vi "Determine Warning Good One.vi"(6 "강풍":dbl, 7 "현재 풍속":dbl, 8 "에러 입력 (에러 없음)":errorcluster caption="에러 입력(에러 없음)", 9 "최저 온도":dbl, 10 "최고 온도":dbl, 11 "현재 온도":dbl) -> (0 "에러 출력":errorcluster, 1 "경고?":bool, 2 "경고 텍스트":string)   [LabVIEW 2010]
doc: "이 VI는 LabVIEW Core II 교육과정의 연습문제에 대한 솔루선입니다. 이 연습문제에서는 물려받은 코드를 읽기 쉽고 유지하기 쉽게 변경합니다."
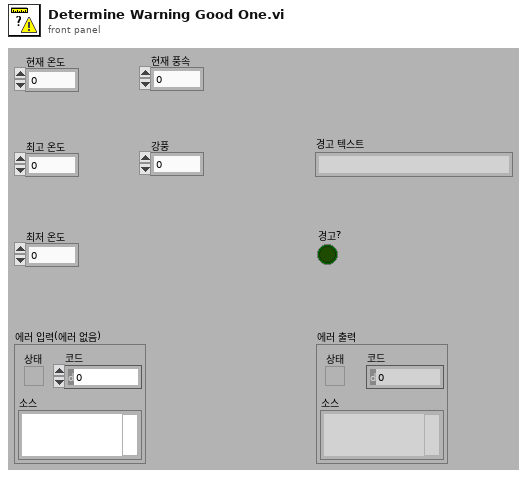
[diagram p1: front panel]
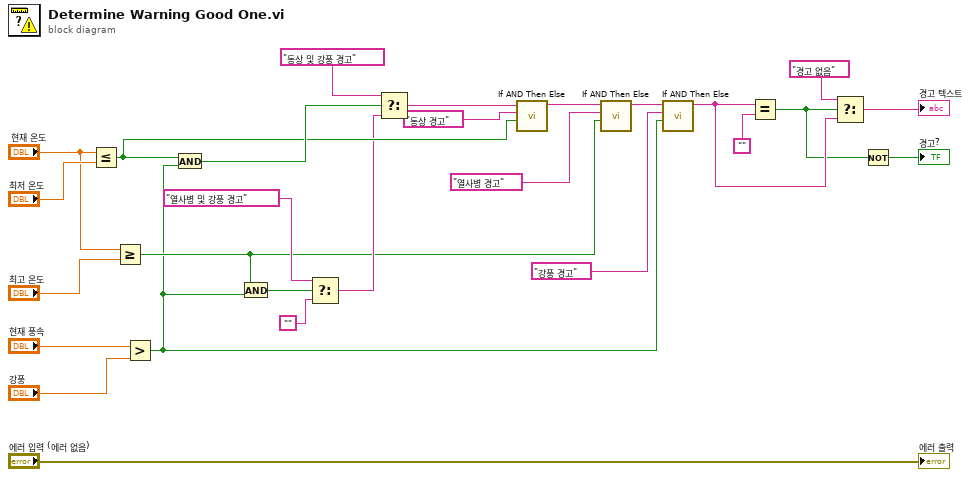
[diagram p0: block diagram]
diagram:
  n1 = Less Or Equal?(x="현재 온도", y="최저 온도") -> (x <= y?=w17:bool)
  n2 = Greater Or Equal?(x="현재 온도", y="최고 온도") -> (x >= y?=w6:bool)
  n3 = Greater?(x="현재 풍속", y="강풍") -> (0:w3:bool)
  n4 = And(x=w17, y=w3) -> (x .and. y?=w18:bool)
  n5 = And(x=w6, y=w3) -> (x .and. y?=w21:bool)
  n6 = Select(t="열사병 및 강풍 경고", s=w21, f="") -> (s? t:f=w15:string)
  n7 = Select(t="동상 및 강풍 경고", s=w18, f=w15) -> (s? t:f=w10:string)
  n8 = call "If AND Then Else.vi"("AND 조건"=w17, "AND 조건 텍스트"="동상 경고", "현재 텍스트"=w10) -> ("현재 텍스트 출력"=w7:string)  [unwired: 6 in]
  n9 = call "If AND Then Else.vi"("AND 조건"=w6, "AND 조건 텍스트"="열사병 경고", "현재 텍스트"=w7) -> ("현재 텍스트 출력"=w4:string)  [unwired: 6 in]
  n10 = call "If AND Then Else.vi"("AND 조건"=w3, "AND 조건 텍스트"="강풍 경고", "현재 텍스트"=w4) -> ("현재 텍스트 출력"=w2:string)  [unwired: 6 in]
  n11 = Equal?(x=w2, y="") -> (x = y?=w1:bool)
  n12 = Select(t="경고 없음" ("f"), s=w1, f=w2) -> (s? t:f=→"경고 텍스트":string)
  n13 = Not(x=w1) -> (.not. x?=→"경고?":bool)
  "에러 출력" <- "에러 입력 (에러 없음)"
